vi "ADAM_scan_table.vi"() -> ()   [LabVIEW 2013]
uses:
  Anemometry/Anemometry Sub Vis/Controls/Serveds.ctl
  ADAM Client/Sub VIs/ADAM Controls/Module_type_ADAM.ctl
  ADAM Client/Sub VIs/ADAM Controls/Traverse_Level_State.ctl
  Anemometry/Anemometry Sub Vis/Controls/Post_Process.ctl
  ADAM Client/Sub VIs/ADAM Controls/Channel_State.ctl
  ADAM Client/Sub VIs/ADAM Controls/Ch_description_ADAM.ctl
  ADAM Client/Sub VIs/ADAM Controls/Function_ADAM.ctl
  ADAM Client/Sub VIs/ADAM Controls/Calib_type_ADAM.ctl
  ADAM Client/Sub VIs/ADAM Controls/Address.ctl
  ADAM_Global.vi
  Sub VI's/Channel_Description_Global.vi
  Anemometry/Anemometry Sub Vis/Globals/Meas_global.vi
  Sub VI's/Logged_Data_real_Global.vi
  Anemometry/Anemometry Sub Vis/Globals/Preference_global.vi
  Anemometry/Anemometry Sub Vis/Globals/Gas_management_global.vi
  Anemometry/Anemometry Sub Vis/Globals/Constants_global.vi
panel:
  in  "Reconfigure Gills":bool
  in  "Full Res Pathname":path
  in  "Log full Res Data":bool
  out "Duty No":u16 format="%.0b"
  in  "Save Current setup":bool=TRUE
  in  "Load setup from file":bool
  out "ADAM scan comments":string
  out "History length":i32=250
  in  "stop":bool
  out "Results":dbl[](array[numeric]) format="%.3f"
  out "Titles":string[](array[string])
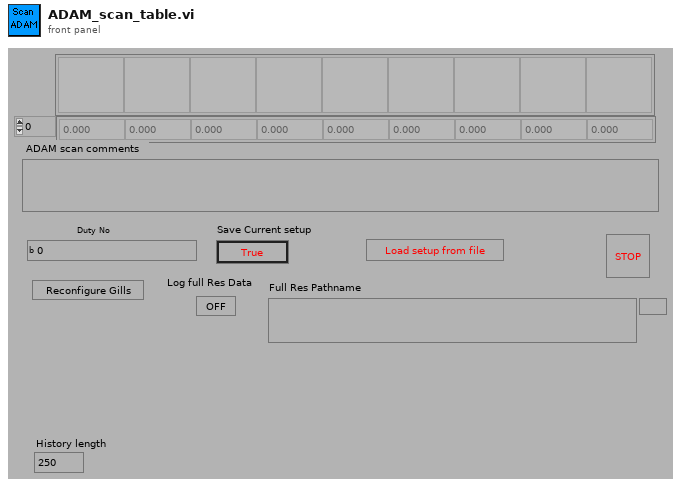
[diagram p1: front panel]
types:
  T1 = enum16{"Load ADAM setup from excel file", "Save ADAM setup to excel file"}
  T2 = typedef "Serveds.ctl" = enum16{"Read Global", "Load Global From File"}
  T3 = typedef "Module_type_ADAM.ctl" = string
  T4 = typedef "Traverse_Level_State.ctl" = enum16{"Running", "Complete"}
  T5 = typedef "Post_Process.ctl" = enum16{"Take New Data", "Post Process Raw Data File"}
  T6 = typedef "Channel_State.ctl" = enum16{"On", "Off", "Always On", "Always Off"}
  T7 = enum16{"Append to Global", "Read Global then Clear"}
  T8 = typedef "Ch_description_ADAM.ctl" = cluster{"Ch Name":string, "Type":T3, "Function":T9, "Ch State":T6, "Calibration type":T10, "A":dbl, "B":dbl, "C":dbl, "D":dbl, "Comments":string, "Address":T11, "String":string, "Duty":u16}
  T9 = typedef "Function_ADAM.ctl" = enum16{"Analogue Input", "Digital Input", "Event counter", "Event rate", "Analogue Output", "Digital Output", "Relay Output"}
  T10 = typedef "Calib_type_ADAM.ctl" = enum16{"Raw", "Bx + A", "Cx^2 + Bx + A", "Dx^3 + Cx^2 + Bx + A", "In Band", "Hi-Tec Q", "Hi-Tec M_dot", "Text"}
  T11 = typedef "Address.ctl" = cluster{"Main":i32, "Ch.":i32, "Sub":i32, "Port Name":string}
  T12 = typedef "Client_State_Cluster.ctl" = cluster{"Client Name":string, "Traverse level State":T4, "People to Email":string[], "Next Contact Time":dbl}
  T13 = typedef "ADAM_Comparitor.ctl" = cluster{"Ch to Monitor":string, "Channels to Kill":string, "Warn if Above":dbl, "Warn if Below":dbl, "Kill if Above":dbl, "Kill if Below":dbl, "Hysteresis Margin":dbl, "Averaging TIme (s)":dbl, "Warn Status":bool, "Kill Status":bool, "Extra Email addresses":string}
  T14 = typedef "Update_scan_value.ctl" = cluster{"Channel Name":string, "New Value":dbl}
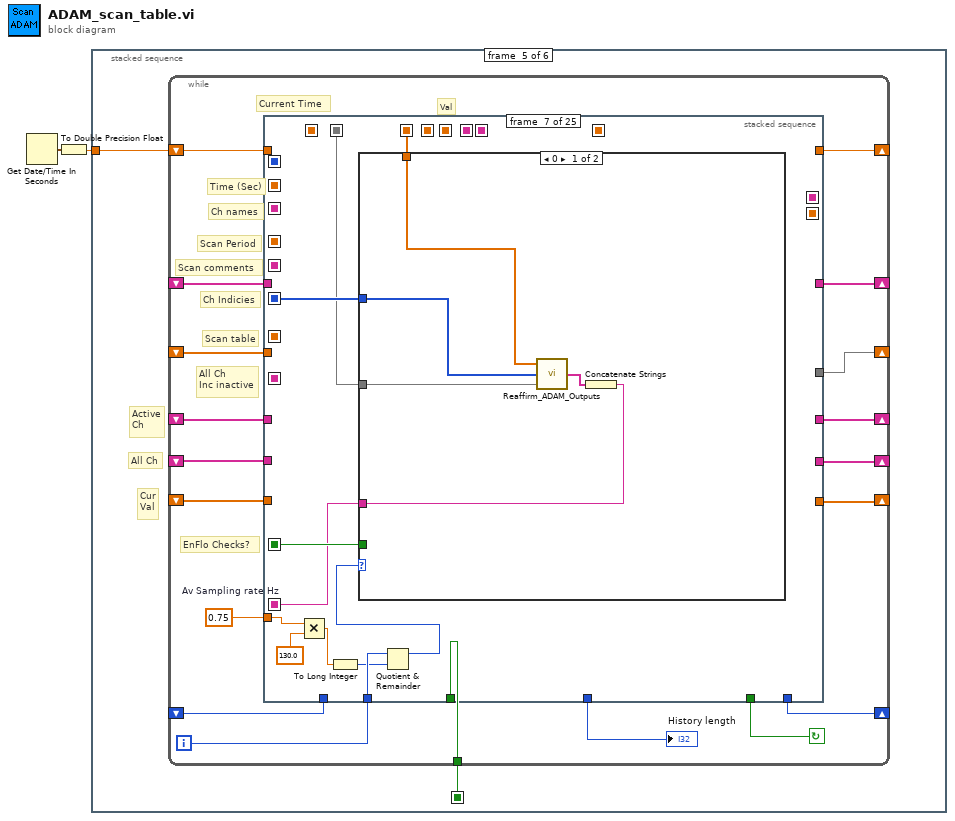
[diagram p0: block diagram]
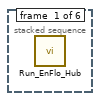
[diagram p2: hidden frame]
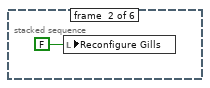
[diagram p3: hidden frame]
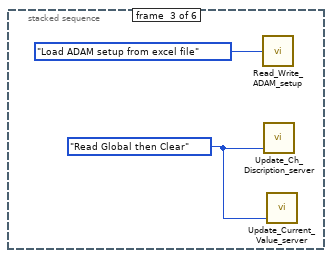
[diagram p4: hidden frame]
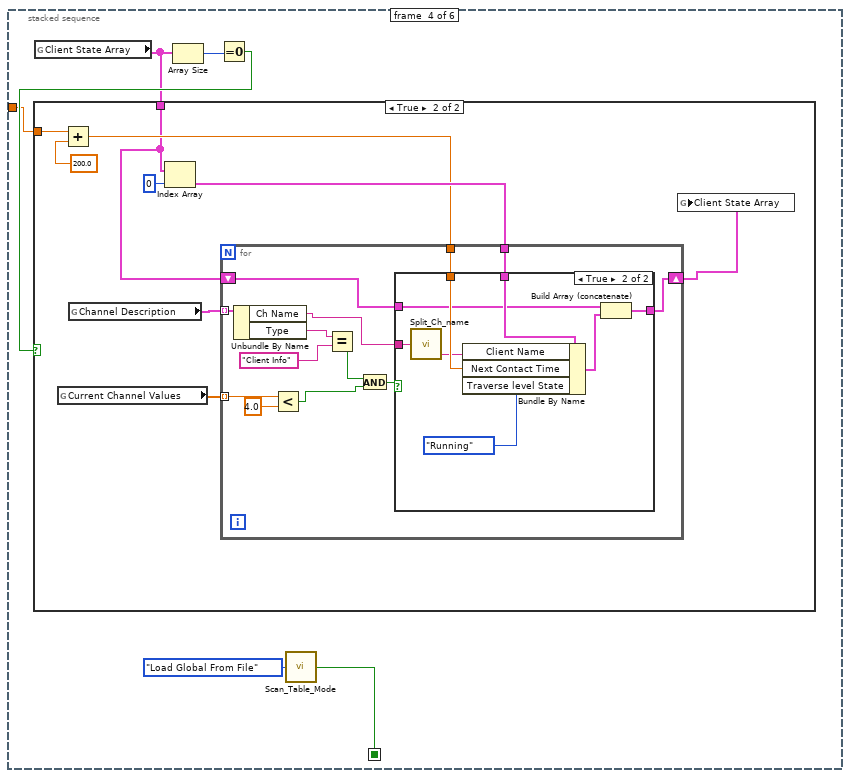
[diagram p5: hidden frame]
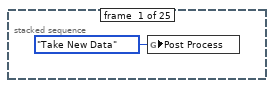
[diagram p8: hidden frame]
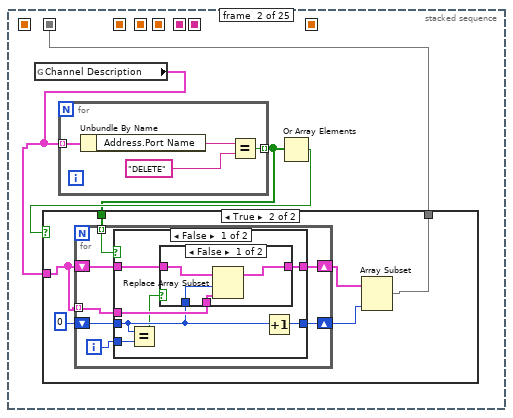
[diagram p9: hidden frame]
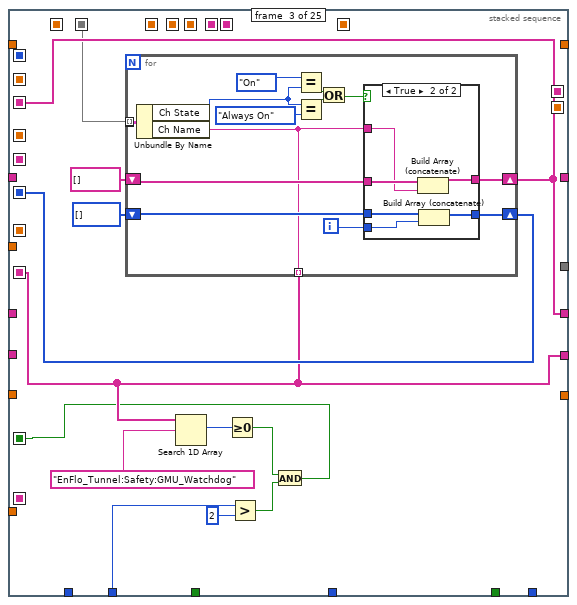
[diagram p13: hidden frame]
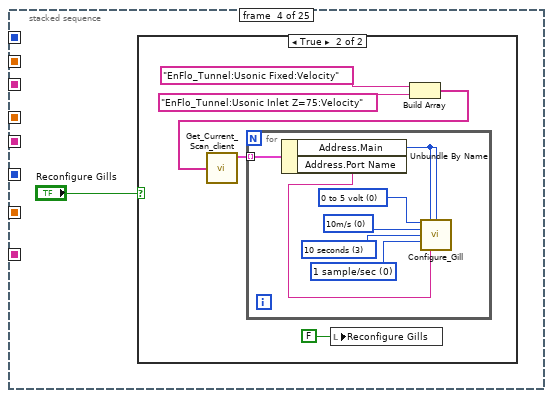
[diagram p15: hidden frame]
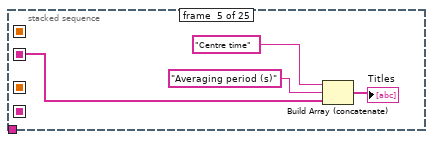
[diagram p17: hidden frame]
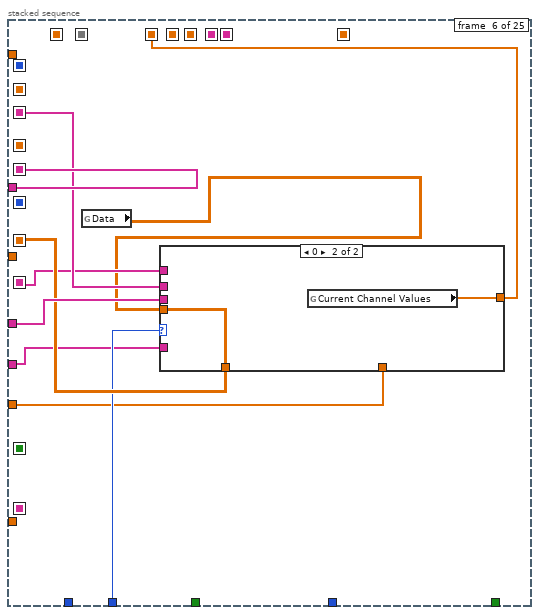
[diagram p18: hidden frame]
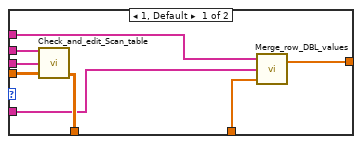
[diagram p19: hidden frame]
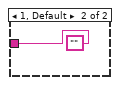
[diagram p20: hidden frame]
diagram:
  n1 = Get Date/Time In Seconds() -> (seconds since 1Jan1904=w2:timestamp)
  n2 = To Double Precision Float(number=w2) -> (double precision float=w1:dbl)
  n3 = stacked-sequence {
    seq-local: [_ _ _ w11 _ _] -> [_ _ _ _ w44 _]
    tunnel: w1 -> [_ _ _ w6 w43 _]
    frame #0 {
      n4 = call "Run_EnFlo_Hub.vi"() -> ()  [unwired: 8 out]
    }
    frame #1 {
      n5 = local write "Reconfigure Gills"(FALSE ("Reconfigure Gills")) -> ()
    }
    frame #2 {
      w4 = T7."Read Global then Clear" ("Mode")
      n6 = call "Read_Write_ADAM_setup.vi"("Mode"=T1."Load ADAM setup from excel file") -> ()  [unwired: 4 out]
      n7 = call "Update_Ch_Discription_server.vi"("Mode"=w4) -> ()  [unwired: 2 in, 1 out]
      n8 = call "Update_Current_Value_server.vi"("Mode"=w4) -> ()  [unwired: 2 in, 1 out]
    }
    frame #3 {
      n9 = global read "ADAM_Global.vi" "Client State Array"() -> (w7:T12[])
      n10 = Array Size(array=w7) -> (size(s)=w9:i32)
      n11 = Equal To 0?(x=w9) -> (x = 0?=w8:bool)
      n12 = case shown="True" w8 {
        tunnel: w7 -> [_ w13]
        tunnel: w6 -> [_ w16]
        frame False {
        }
        frame True {
          n13 = global read "ADAM_Global.vi" "Current Channel Values"() -> (w20:dbl[])
          n14 = Add(x=w16, y=200.0) -> (x+y=w14:dbl)
          n15 = global read "Channel_Description_Global.vi" "Channel Description"() -> (w19:T8[])
          n16 = Index Array(array=w13, index=0) -> (element=w17:T12)
          n17 = for {
            tunnel: w19 -> [w33] mode=indexing
            tunnel: w20 -> [w25] mode=indexing
            tunnel: w17 -> [w26]
            tunnel: w14 -> [w24]
            shift-right: [w23] -> w12
            shift-left: w13 -> [w22]
            n18 = Unbundle By Name(w33) -> ("Ch Name"=w21:string, "Type"=w30:T3)
            n19 = Less?(x=w25, y=4.0) -> (x < y?=w28:bool)
            n20 = Equal?(x=w30, y=T3 "Client Info" ("Type")) -> (x = y?=w29:bool)
            n21 = And(x=w29, y=w28) -> (x .and. y?=w27:bool)
            n22 = case shown="True" w27 {
              tunnel: w26 -> [_ w42]
              tunnel: w24 -> [_ w41]
              tunnel: [w34 w39] -> w23
              tunnel: w22 -> [w34 w38]
              tunnel: w21 -> [_ w36]
              frame False {
              }
              frame True {
                n23 = call "Split_Ch_name.vi"("Ch name"=w36) -> ("Low level"=w35:string)  [unwired: 2 out]
                n24 = Bundle By Name(cluster=w42, "Client Name"=w35, "Next Contact Time"=w41, "Traverse level State"=Traverse_Level_State."Running") -> (w37:T12)
                n25 = Build Array (concatenate)(w38, w37) -> (w39:T12[])
              }
            }
          }
          n26 = global write "ADAM_Global.vi" "Client State Array"(w12) -> ()
        }
      }
      n27 = call "Scan_Table_Mode.vi"("Mode"=Serveds."Load Global From File") -> ("Simulate Mode ?"=w11:bool)
    }
    frame #4 {
      # "Active\nCh"
      # "Cur\nVal"
      # "All Ch"
      n28 = while {
        shift-left: _ -> [w47]
        shift-right: [w46] -> _
        shift-left: _ -> [w48]
        shift-right: [w49] -> _
        shift-left: _ -> [w50]
        shift-right: [w51] -> _
        tunnel: w44 -> [w52]
        shift-left: _ -> [w55]
        shift-right: [w54] -> _
        shift-left: _ -> [w57]
        shift-right: [w58] -> _
        shift-left: _ -> [w59]
        shift-right: [w60] -> _
        shift-left: w43 -> [w61]
        shift-right: [w62] -> _
        i -> [w56]
        stop <- w63 continue-if-true
        w45 = 0.75  # Av Sampling rate Hz
        # "Current Time"
        # "EnFlo Checks?"
        # "Val"
        # "All Ch\nInc inactive"
        # "Scan comments"
        # "Scan table"
        # "Time (Sec)"
        # "Ch Indicies"
        # "Ch names"
        # "Scan Period"
        n29 = stacked-sequence {
          seq-local: [_ _ _ _ _ _ _ _ _ _ _ _ _ _ _ w315 _ _ _ _ _ _ _ _ _] -> [_ _ _ _ _ _ _ _ _ _ _ _ _ _ _ _ _ w366 w371 _ _ _ _ w449 _]
          seq-local: [_ _ _ _ _ _ _ _ w199 _ _ _ _ _ _ _ _ _ _ _ _ _ _ _ _] -> [_ _ _ _ _ _ _ _ _ _ _ _ _ _ _ _ _ _ w378 _ _ _ _ _ _]
          seq-local: [_ _ _ _ _ w158 _ _ _ _ _ _ _ _ _ _ _ _ _ _ _ _ _ _ _] -> [_ _ _ _ _ _ _ w192 _ _ _ _ _ _ _ _ _ _ w376 _ _ _ _ _ _]
          seq-local: [_ _ _ _ _ _ _ _ w203 _ _ _ _ _ _ _ _ _ _ _ _ _ _ _ _] -> [_ _ _ _ _ _ _ _ _ _ w226 _ _ _ _ _ _ _ w377 _ _ _ _ _ _]
          seq-local: [_ _ _ _ _ w161 _ _ _ _ _ _ _ _ _ _ _ _ _ _ _ _ _ _ _] -> [_ _ _ _ _ _ _ w194 _ _ _ _ _ _ _ _ _ _ _ _ w416 _ _ _ _]
          seq-local: [_ _ _ _ _ _ _ _ _ _ w224 _ _ _ _ _ _ _ _ _ _ _ _ _ _] -> [_ _ _ _ _ _ _ _ _ _ _ w243 _ _ _ _ _ _ _ _ _ _ _ _ _]
          seq-local: [_ _ w112 _ _ _ _ _ _ _ _ _ _ _ _ _ _ _ _ _ _ _ _ _ _] -> [_ _ _ _ w150 w160 _ w195 w204 _ _ _ _ _ _ _ _ _ w374 w379 _ _ _ _ _]
          seq-local: [_ _ w111 _ _ _ _ _ _ _ _ _ _ _ _ _ _ _ _ _ _ _ _ _ _] -> [_ _ _ _ _ _ w175 w190 _ _ w225 _ _ _ _ _ _ _ _ _ _ _ _ _ _]
          seq-local: [_ _ _ _ _ w154 _ _ _ _ _ _ _ _ _ _ _ _ _ _ _ _ _ _ _] -> [_ _ _ _ _ _ w173 w191 _ _ w222 _ _ _ _ _ _ _ _ _ _ _ _ _ _]
          seq-local: [_ _ _ _ _ _ _ _ _ _ w220 _ _ _ _ _ _ _ _ _ _ _ _ _ _] -> [_ _ _ _ _ _ _ _ _ _ _ w248 w277 _ _ w313 _ _ _ _ _ _ _ _ _]
          seq-local: [_ _ w107 _ _ _ _ _ _ _ _ _ _ _ _ _ _ _ _ _ _ _ _ _ _] -> [_ _ _ _ _ w156 _ w193 _ _ w221 w247 w276 _ _ w314 w339 w358 w373 _ _ _ w426 _ _]
          seq-local: [_ _ _ _ _ _ _ _ _ w206 _ _ _ _ _ _ _ _ _ _ _ _ _ _ _] -> [_ _ _ _ _ _ _ _ _ _ w219 _ _ _ _ _ _ _ _ _ _ _ _ _ _]
          seq-local: [_ w65 _ _ _ _ _ _ _ _ _ _ _ _ _ _ _ _ _ _ _ _ _ _ _] -> [_ _ w109 _ _ _ w174 w189 _ _ w218 _ _ _ _ _ _ _ _ _ _ _ _ _ _]
          seq-local: [_ _ _ _ _ _ _ _ w198 _ _ _ _ _ _ _ _ _ _ _ _ _ _ _ _] -> [_ _ _ _ _ _ _ _ _ _ _ w244 _ _ _ _ _ _ _ w381 _ _ _ _ _]
          seq-local: [_ _ _ _ _ _ _ _ _ _ _ _ _ _ _ _ _ _ w370 _ _ _ _ _ _] -> [_ _ _ _ _ _ _ _ _ _ _ _ _ _ _ _ _ _ _ w380 _ _ _ _ _]
          seq-local: [_ _ w101 _ _ _ _ _ _ _ _ _ _ _ _ _ _ _ _ _ _ _ _ _ _] -> [_ _ _ _ _ _ w182 _ w196 _ _ w246 w275 w290 w299 _ _ _ _ _ _ _ _ _ w453]
          seq-local: [_ _ _ _ _ _ _ _ _ _ _ _ _ _ _ w312 _ _ _ _ _ _ _ _ _] -> [_ _ _ _ _ _ _ _ _ _ _ _ _ _ _ _ w340 _ _ _ _ _ _ _ _]
          seq-local: [_ _ _ _ _ _ w172 _ _ _ _ _ _ _ _ _ _ _ _ _ _ _ _ _ _] -> [_ _ _ _ _ _ _ _ _ _ w217 _ _ _ _ _ _ _ _ _ _ _ _ _ _]
          seq-local: [_ _ _ _ _ _ _ _ _ _ _ _ _ _ _ w311 _ _ _ _ _ _ _ _ _] -> [_ _ _ _ _ _ _ _ _ _ _ _ _ _ _ _ w338 _ _ _ _ _ _ _ _]
          seq-local: [_ _ _ _ _ _ _ _ _ _ _ w242 _ _ _ _ _ _ _ _ _ _ _ _ _] -> [_ _ _ _ _ _ _ _ _ _ _ _ _ _ _ _ _ _ _ _ w404 _ _ _ _]
          tunnel: [_ _ _ _ _ _ _ _ _ _ _ _ _ _ _ _ _ _ _ _ _ w424 _ _ _] -> w63
          tunnel: [_ _ _ _ _ _ _ _ w198 _ _ _ _ _ _ _ _ _ _ _ _ _ _ _ _] -> w62
          tunnel: w61 -> [_ _ _ _ _ _ _ _ w200 _ _ _ _ _ _ _ _ _ _ _ _ _ _ _ _]
          tunnel: [_ _ _ _ _ _ _ _ _ _ _ _ _ _ _ _ _ _ _ _ w414 _ _ _ _] -> w60
          tunnel: w59 -> [_ _ _ _ _ w161 _ _ _ _ _ _ _ _ _ _ _ _ _ _ _ _ _ _ _]
          tunnel: [_ _ w112 _ _ _ _ _ _ _ _ _ _ _ _ _ _ _ _ _ _ _ _ _ _] -> w58
          tunnel: w57 -> [_ _ _ _ _ w159 _ _ _ _ _ _ _ _ _ _ w341 _ _ _ _ _ _ _ _]
          tunnel: w56 -> [_ _ w105 _ _ w157 w178 _ _ _ _ w245 w271 w286 w295 _ _ _ _ _ _ w422 _ _ w454]
          tunnel: w55 -> [_ _ _ _ _ _ _ _ _ _ _ _ _ _ _ _ _ w364 _ _ _ _ _ _ _]
          tunnel: [_ _ _ _ _ _ _ _ _ _ _ _ _ _ _ _ _ w360 _ _ _ _ _ _ _] -> w54
          tunnel: [_ _ _ _ _ _ _ _ _ _ _ _ _ _ _ _ _ _ w375 _ _ _ _ _ _] -> w53
          tunnel: w52 -> [_ _ _ _ _ _ _ _ _ _ w223 _ _ _ _ _ _ _ _ _ _ _ _ _ _]
          tunnel: [_ _ w107 _ _ _ _ _ _ _ _ _ _ _ _ _ _ _ _ _ _ _ _ _ _] -> w51
          tunnel: w50 -> [_ _ _ _ _ w155 _ _ _ _ _ _ _ _ _ _ _ _ _ _ _ _ _ _ _]
          tunnel: [_ _ _ _ _ _ _ _ _ _ _ _ _ _ _ _ _ _ _ _ _ _ _ w449 _] -> w49
          tunnel: w48 -> [_ _ _ _ _ w153 _ _ _ _ _ _ _ _ _ _ _ _ _ _ _ _ _ _ _]
          tunnel: w47 -> [_ _ _ _ _ _ _ _ _ w207 _ _ _ _ _ _ _ _ _ _ _ _ _ _ _]
          tunnel: [_ _ _ _ _ _ _ _ _ w208 _ _ _ _ _ _ _ _ _ _ _ _ _ _ _] -> w46
          tunnel: w45 -> [_ _ _ _ _ _ w181 _ _ _ _ _ w274 w289 w298 _ _ _ _ _ _ _ _ _ _]
          frame #0 {
            n30 = global write "Meas_global.vi" "Post Process"(Post_Process."Take New Data" ("Post Process")) -> ()
          }
          frame #1 {
            n31 = global read "Channel_Description_Global.vi" "Channel Description"() -> (w67:T8[])
            n32 = for {
              tunnel: w67 -> [w100] mode=indexing
              tunnel: [w97] -> w66 mode=indexing
              n33 = Unbundle By Name(w100) -> ("Address.Port Name"=w99:string)
              n34 = Equal?(x=w99, y="DELETE") -> (x = y?=w97:bool)
            }
            n35 = Or Array Elements(Boolean array=w66) -> (logical OR=w68:bool)
            n36 = case shown="True" w68 {
              tunnel: w67 -> [w69 w73]
              tunnel: w66 -> [_ w75]
              tunnel: [w69 w70] -> w65
              frame False {
              }
              frame True {
                n37 = for {
                  shift-right: [w82] -> w72
                  shift-left: w73 -> [w81]
                  tunnel: w75 -> [w77] mode=indexing
                  shift-right: [w80] -> w71
                  shift-left: 0 -> [w78]
                  tunnel: w73 -> [w79] mode=indexing
                  i -> [w76]
                  n38 = case shown="False" w77 {
                    tunnel: [w88 w96] -> w82
                    tunnel: w81 -> [w89 w96]
                    tunnel: [w86 w95] -> w80
                    tunnel: w78 -> [w85 w95]
                    tunnel: w79 -> [w87 _]
                    tunnel: w76 -> [w84 _]
                    frame False {
                      n39 = Equal?(x=w85, y=w84) -> (x = y?=w83:bool)
                      n40 = case shown="False" w83 {
                        tunnel: w89 -> [w93 w94]
                        tunnel: [w92 w94] -> w88
                        tunnel: w87 -> [w91 _]
                        tunnel: w85 -> [w90 _]
                        frame False {
                          n41 = Replace Array Subset(array=w93, new element=w91, index=w90) -> (w92:T8[])
                        }
                        frame True {
                        }
                      }
                      n42 = Increment(x=w85) -> (x+1=w86:i32)
                    }
                    frame True {
                    }
                  }
                }
                n43 = Array Subset(array=w72, length=w71) -> (w70:T8[])  [unwired: 1 in]
              }
            }
          }
          frame #2 {
            n44 = for {
              tunnel: [w126] -> _ mode=indexing
              shift-right: [w125] -> w112
              shift-left: string[] [] -> [w116]
              shift-right: [w122] -> w111
              shift-left: i32[] [] -> [w124]
              tunnel: [w114] -> w107 mode=indexing
              tunnel: w109 -> [w126] mode=indexing
              i -> [w123]
              n45 = Unbundle By Name(w126) -> ("Ch State"=w117:T6, "Ch Name"=w114:string)
              n46 = Equal?(x=Channel_State."On" ("Channel State"), y=w117) -> (x = y?=w119:bool)
              n47 = Equal?(x=w117, y=Channel_State."Always On" ("Channel State")) -> (x = y?=w118:bool)
              n48 = Or(x=w119, y=w118) -> (x .or. y?=w115:bool)
              n49 = case shown="True" w115 {
                tunnel: w116 -> [w127 w134]
                tunnel: w114 -> [_ w133]
                tunnel: [w127 w132] -> w125
                tunnel: w124 -> [w128 w131]
                tunnel: w123 -> [_ w130]
                tunnel: [w128 w129] -> w122
                frame False {
                }
                frame True {
                  n50 = Build Array (concatenate)(w134, w133) -> (w132:string[])
                  n51 = Build Array (concatenate)(w131, w130) -> (w129:i32[])
                }
              }
            }
            n52 = Search 1D Array(1D array=w107, element="EnFlo_Tunnel:Safety:GMU_Watchdog") -> (index of element=w106:i32)  [unwired: 1 out]
            n53 = Greater Or Equal To 0?(x=w106) -> (x >= 0?=w102:bool)
            n54 = Greater?(x=w105, y=2) -> (0:w103:bool)
            n55 = And(x=w102, y=w103) -> (x .and. y?=w101:bool)
          }
          frame #3 {
            n56 = case shown="True" "Reconfigure Gills" {
              frame False {
              }
              frame True {
                n57 = local write "Reconfigure Gills"(FALSE ("Reconfigure Gills")) -> ()
                n58 = Build Array("EnFlo_Tunnel:Usonic Fixed:Velocity", "EnFlo_Tunnel:Usonic Inlet Z=75:Velocity") -> (w138:string[])
                n59 = call "Get_Current_Scan_client.vi"("ADAM Ch Names"=w138) -> ("Ch Description Array"=w137:T8[])  [unwired: 3 out]
                n60 = for {
                  tunnel: w137 -> [w143] mode=indexing
                  w147 = u16 0 items=["1 sample/sec", "4 samples/sec"] ("Samples/sec")
                  w146 = u16 3 items=["OFF", "3 seconds", "5 seconds", "10 seconds"] ("Averaging Time")
                  w145 = u16 0 items=["10m/s", "20m/s", "30m/s", "40m/s", "50m/s", "60m/s", "70m/s"] ("Analogue O/P Scale")
                  w144 = u16 0 items=["0 to 5 volt", "+/-2.5 Volt", "4-20mA"] ("Analogue O/P Config")
                  n61 = Unbundle By Name(w143) -> ("Address.Main"=w142:i32, "Address.Port Name"=w141:string)
                  n62 = call "Configure_Gill.vi"("Analogue O/P Config"=w144, "ORIGINAL Address"=w142, "NEW Address"=w142, "Analogue O/P Scale"=w145, "Averaging Time"=w146, "Samples/sec"=w147, "Port Name"=w141) -> ()  [unwired: 9 out]
                }
              }
            }
          }
          frame #4 {
            n63 = Build Array (concatenate)("Centre time", "Averaging period (s)", w150) -> (→"Titles":string[])
          }
          frame #5 {
            n64 = global read "Logged_Data_real_Global.vi" "Data"() -> (w152:dbl[][])
            n65 = case shown="0" w157 {
              tunnel: w152 -> [w169 w171]
              tunnel: w160 -> [w166 _]
              tunnel: w159 -> [w168 _]
              tunnel: [w167 w171] -> w158
              tunnel: w156 -> [w165 _]
              tunnel: w155 -> [w164 _]
              tunnel: [w163 w170] -> w154
              tunnel: w153 -> [w162 _]
              frame 1, Default {
                n66 = call "Check_and_edit_Scan_table.vi"("2D array input"=w169, "Original Channels"=w168, "Present Channels"=w166) -> ("2D array output"=w167:dbl[][])  [unwired: 2 out]
                n67 = call "Merge_row_DBL_values.vi"("Present Row values"=w162, "Present Channels"=w164, "Desired Channels"=w165) -> ("Desired Row values"=w163:dbl[])  [unwired: 1 out]
              }
              frame 0 {
                n68 = global read "ADAM_Global.vi" "Current Channel Values"() -> (w170:dbl[])
              }
            }
          }
          frame #6 {
            n69 = Multiply(x=w181, y=130.0) -> (x*y=w179:dbl)
            n70 = To Long Integer(number=w179) -> (32bit integer=w177:i32)
            n71 = Quotient & Remainder(x=w178, y=w177) -> (x-y*floor(x/y)=w176:i32)  [unwired: 1 out]
            n72 = case shown="0" w176 {
              tunnel: w182 -> [_ _]
              tunnel: w175 -> [w186 _]
              tunnel: w174 -> [w185 _]
              tunnel: w173 -> [w184 _]
              tunnel: [w183 ""] -> w172
              frame 0 {
                n73 = call "Reaffirm_ADAM_Outputs.vi"("Channel Description"=w185, "Active Ch Indicies"=w186, "Current Channel Values"=w184) -> ("Scan Comments"=w187:string[])  [unwired: 2 out]
                n74 = Concatenate Strings(w187) -> (w183:string)
              }
              frame 1, Default {
              }
            }
          }
          frame #7 {
            n75 = global write "ADAM_Global.vi" "Active Ch names"(w195) -> ()
            n76 = global write "ADAM_Global.vi" "Scan comments"(w194) -> ()
            n77 = global write "Channel_Description_Global.vi" "Channel Description"(w189) -> ()
            n78 = global write "ADAM_Global.vi" "Active Ch Indicies"(w190) -> ()
            n79 = global write "ADAM_Global.vi" "All Ch names"(w193) -> ()
            n80 = global write "Logged_Data_real_Global.vi" "Data"(w192) -> ()
            n81 = global write "ADAM_Global.vi" "Current Channel Values"(w191) -> ()
          }
          frame #8 {
            n82 = case shown="True" w196 {
              tunnel: w204 -> [_ w205]
              frame False {
              }
              frame True {
                n83 = call "Gas_Status_panel.vi"("Ch names"=w205) -> ()  [unwired: 15 out]
              }
            }
            n84 = Get Date/Time In Seconds() -> (seconds since 1Jan1904=w197:timestamp)
            n85 = To Double Precision Float(number=w197) -> (double precision float=w198:dbl)
            n86 = Subtract(x=w198, y=w200) -> (x-y=w203:dbl)
            n87 = Divide(x=w203, y=2.0) -> (x/y=w201:dbl)
            n88 = Add(x=w201, y=w200) -> (x+y=w199:dbl)
          }
          frame #9 {
            n89 = Equal To 0?(x=w207) -> (x = 0?=w211:bool)
            n90 = Equal?(x=u16 32768, y=w207) -> (x = y?=w210:bool)
            n91 = Select(t=u16 1, s=w211, f=w207) -> (s? t:f=w206:u16)
            "Duty No" <- w206
            n92 = case shown="False" w210 {
              tunnel: [w213 u16 0] -> w208
              tunnel: w206 -> [w215 _]
              frame False {
                n93 = Multiply(x=u16 2, y=w215) -> (x*y=w213:u16)
              }
              frame True {
              }
            }
          }
          frame #10 {
            n94 = for {
              tunnel: w218 -> [w233]
              tunnel: w226 -> [w241]
              shift-right: [w239] -> w220
              shift-left: w222 -> [w237]
              tunnel: w221 -> [w238]
              shift-right: [w234] -> w224
              shift-left: w217 -> [w236]
              tunnel: w225 -> [w228] mode=indexing
              tunnel: w222 -> [w230]
              tunnel: w223 -> [w231]
              tunnel: w219 -> [w227]
              n95 = Index Array(array=w230, index=w228) -> (element=w229:dbl)
              n96 = Index Array(array=w233, index=w228) -> (element=w232:T8)
              n97 = call "Adam_Ch_Input_Output.vi"("Simulate"=w231, "Duty No"=w227, "Previuos Scan Value"=w229, "Ch values"=w237, "Scan Period"=w241, "Ch Discription"=w232, "Ch names"=w238) -> ("Scan comment"=w235:string, "Calibrated units"=w240:dbl)  [unwired: 1 in, 2 out]
              n98 = Concatenate Strings(w236, w235) -> (w234:string)
              n99 = Replace Array Subset(array=w237, new element=w240, index=w228) -> (w239:dbl[])
            }
          }
          frame #11 {
            n100 = case shown="True" w246 {
              tunnel: w248 -> [_ w255]
              tunnel: w247 -> [_ w254]
              tunnel: w245 -> [_ w253]
              tunnel: w244 -> [_ w263]
              tunnel: w243 -> [w250 w252]
              tunnel: [w250 w260] -> w242
              frame False {
              }
              frame True {
                n101 = global read "ADAM_Global.vi" "Comparitor Array"() -> (w259:T13[])
                n102 = for {
                  tunnel: w259 -> [w268] mode=indexing
                  tunnel: [w267] -> w258 mode=indexing
                  tunnel: w255 -> [w266]
                  tunnel: w254 -> [w265]
                  tunnel: [w264] -> w257 mode=indexing
                  n103 = call "ADAM_Comparitor.vi"("Comparator Info"=w268, "Ch names"=w265, "Present scan array"=w266) -> ("Comparator Info Out"=w267:T13, "Scan comment"=w264:string)  [unwired: 1 in]
                }
                n104 = call "LDA1_Safety.vi"("Adam Loop Count"=w253, "Ch Names"=w254, "Values"=w255) -> ("Scan comment"=w251:string)
                n105 = call "LDA2_Safety.vi"("Adam Loop Count"=w253, "Ch Names"=w254, "Values"=w255) -> ("Scan comment"=w256:string)
                n106 = call "Safety_Check.vi"("Adam Loop Count"=w253, "Ch Names"=w254, "Values"=w255) -> ("Scan comment"=w262:string)
                n107 = call "Check_Aero_Tunnel_on_Server.vi"("Values"=w255, "Ch Names"=w254, "Current Time"=w263, "Adam Loop Count"=w253) -> ("Scan comment"=w261:string)  [unwired: 2 in]
                n108 = global write "ADAM_Global.vi" "Comparitor Array"(w258) -> ()
                n109 = Concatenate Strings(w252, w251, w256, w262, w261, w257) -> (w260:string)
              }
            }
            n110 = property on="Results" class="Arr (strict)"() -> ("Index Values"=w249:u32[])  [unwired: 2 in, 2 out]
            n111 = property on="Titles" class="Arr (strict)"("Index Values"=w249) -> ()  [unwired: 2 in, 2 out]
          }
          frame #12 {
            n112 = Multiply(x=w274, y=60.0) -> (x*y=w272:dbl)
            n113 = To Long Integer(number=w272) -> (32bit integer=w270:i32)
            n114 = Quotient & Remainder(x=w271, y=w270) -> (x-y*floor(x/y)=w269:i32)  [unwired: 1 out]
            n115 = case shown="0" w269 {
              tunnel: w277 -> [w280 _]
              tunnel: w276 -> [w279 _]
              tunnel: w275 -> [w278 _]
              frame 0 {
                n116 = case shown="True" w278 {
                  tunnel: w280 -> [_ w283]
                  tunnel: w279 -> [_ w282]
                  frame False {
                  }
                  frame True {
                    w281 = TRUE  # Set Watchdogs
                    n117 = call "Do_Every_minute.vi"("Ch Names"=w282, "Values"=w283) -> ()  [unwired: 1 out]
                    n118 = call "Set_Adam_Watchdogs.vi"("Set Watchdogs"=w281) -> ()  [unwired: 1 out]
                  }
                }
              }
              frame 1, Default {
              }
            }
          }
          frame #13 {
            n119 = Multiply(x=w289, y=100.0) -> (x*y=w287:dbl)
            n120 = To Long Integer(number=w287) -> (32bit integer=w285:i32)
            n121 = Quotient & Remainder(x=w286, y=w285) -> (x-y*floor(x/y)=w284:i32)  [unwired: 1 out]
            n122 = case shown="0" w284 {
              tunnel: w290 -> [w291 _]
              frame 0 {
                n123 = case shown="True" w291 {
                  frame False {
                  }
                  frame True {
                    w292 = TRUE  # Set Watchdogs
                    n124 = call "Set_Adam_Watchdogs.vi"("Set Watchdogs"=w292) -> ()  [unwired: 1 out]
                  }
                }
              }
              frame 1, Default {
              }
            }
          }
          frame #14 {
            n125 = Multiply(x=w298, y=55.0) -> (x*y=w296:dbl)
            n126 = To Long Integer(number=w296) -> (32bit integer=w294:i32)
            n127 = Quotient & Remainder(x=w295, y=w294) -> (x-y*floor(x/y)=w293:i32)  [unwired: 1 out]
            n128 = case shown="0" w293 {
              tunnel: w299 -> [_ _]
              frame 0 {
                n129 = case shown="True" "Save Current setup" {
                  tunnel: [FALSE w303] -> w300
                  frame False {
                  }
                  frame True {
                    n130 = Get Date/Time In Seconds() -> (seconds since 1Jan1904=w305:timestamp)
                    n131 = global read "ADAM_Global.vi" "Network Last checked"() -> (w309:dbl)
                    n132 = To Double Precision Float(number=w305) -> (double precision float=w304:dbl)
                    n133 = Subtract(x=w309, y=w304) -> (x-y=w308:dbl)
                    n134 = Absolute Value(x=w308) -> (abs(x)=w307:dbl)
                    n135 = Less?(x=w307, y=1.5) -> (x < y?=w303:bool)
                  }
                }
                n136 = case shown="True" w300 {
                  frame False {
                  }
                  frame True {
                    n137 = call "Read_Write_ADAM_setup.vi"("Mode"=T1."Save ADAM setup to excel file") -> ()  [unwired: 4 out]
                  }
                }
              }
              frame 1, Default {
              }
            }
          }
          frame #15 {
            n138 = call "Update_Current_Value_server.vi"("Mode"=T7."Read Global then Clear") -> ("Update array out"=w317:T14[])  [unwired: 2 in]
            n139 = for {
              tunnel: w314 -> [w325]
              tunnel: w317 -> [w320] mode=indexing
              shift-right: [w323] -> w315
              shift-left: w313 -> [w324]
              tunnel: [w319] -> w312 mode=indexing
              tunnel: [w318] -> w311 mode=indexing
              n140 = Unbundle By Name(w320) -> ("Channel Name"=w319:string, "New Value"=w318:dbl)
              n141 = Search 1D Array(1D array=w325, element=w319) -> (index of element=w322:i32)  [unwired: 1 out]
              n142 = Less Than 0?(x=w322) -> (x < 0?=w321:bool)
              n143 = case shown="True" w321 {
                tunnel: w319 -> [_ w326]
                tunnel: w320 -> [_ w331]
                frame False {
                }
                frame True {
                  n144 = global read "ADAM_Global.vi" "Update Current Value"() -> (w330:T14[])
                  n145 = call "Check_Ch_Name_colons.vi"("No of Colons"=2, "Ch Name in"=w326) -> ("Ch Name out"=w327:string)
                  n146 = Bundle By Name(cluster=T8 {"Ch Name"="", "Type"="Hold Value", "Function"=enum."Analogue Input", "Ch State"=enum."On", "Calibration type"=enum."Raw", "A"=0.0, "B"=0.0, "C"=0.0, "D"=0.0, "Comments"="", "Address"={"Main"=0, "Ch."=0, "Sub"=0, "Port Name"=""}, "String"="", "Duty"=0} ("Ch Description"), "Ch Name"=w327, "Type"=T3 "Hold Value") -> (w335:T8)
                  n147 = Build Array (concatenate)(w330, w331) -> (w329:T14[])
                  n148 = global write "ADAM_Global.vi" "Update Current Value"(w329) -> ()
                  n149 = global read "Preference_global.vi" "Rig Setup"() -> (w333:string)
                  n150 = Build Array(w335) -> (w334:T8[])
                  n151 = call "Update_Ch_Discription_server.vi"("Mode"=T7."Append to Global", "Client HD name"=w333, "Channels to update In"=w334) -> ()  [unwired: 1 out]
                }
              }
              n152 = Replace Array Subset(array=w324, new element=w318, index=w322) -> (w323:dbl[])
            }
          }
          frame #16 {
            n153 = for {
              tunnel: w341 -> [w349]
              tunnel: w340 -> [w347] mode=indexing
              tunnel: w339 -> [w348]
              tunnel: w338 -> [w345] mode=indexing
              n154 = Search 1D Array(1D array=w349, element=w347) -> (index of element=w346:i32)  [unwired: 1 out]
              n155 = Less Than 0?(x=w346) -> (x < 0?=w344:bool)
              n156 = Not Equal To 0?(x=w345) -> (x != 0?=w343:bool)
              n157 = And(x=w343, y=w344) -> (x .and. y?=w342:bool)
              n158 = case shown="True" w342 {
                tunnel: w348 -> [_ w357]
                tunnel: w347 -> [_ w356]
                frame False {
                }
                frame True {
                  n159 = Search 1D Array(1D array=w357, element=w356) -> (index of element=w351:i32)  [unwired: 1 out]
                  n160 = global read "Channel_Description_Global.vi" "Channel Description"() -> (w352:T8[])
                  n161 = Index Array(array=w352, index=w351) -> (element=w355:T8)
                  n162 = Bundle By Name(cluster=w355, "Ch State"=Channel_State."On") -> (w353:T8)
                  n163 = Replace Array Subset(array=w352, new element=w353, index=w351) -> (w350:T8[])
                  n164 = global write "Channel_Description_Global.vi" "Channel Description"(w350) -> ()
                }
              }
            }
          }
          frame #17 {
            n165 = Search 1D Array(1D array=w358, element="GMU:Source:Release Temp") -> (index of element=w365:i32)  [unwired: 1 out]
            n166 = Index Array(array=w366, index=w365) -> (element=w363:dbl)
            n167 = Build Array (concatenate)(w363, w364) -> (w362:dbl[])
            n168 = Array Subset(array=w362, length=10 ("Array Length")) -> (w360:dbl[])  [unwired: 1 in]
            n169 = call "Mean_fr_NaN_data.vi"("Data"=w360) -> ("Mean value"=w359:dbl)  [unwired: 1 out]
            n170 = global write "Gas_management_global.vi" "Release temp (deg C)"(w359) -> ()
          }
          frame #18 {
            w368 = 250000  # Table size
            n171 = call "Merge_row_DBL_values.vi"("Present Row values"=w371, "Present Channels"=w373, "Desired Channels"=w374) -> ("Desired Row values"=w372:dbl[])  [unwired: 1 out]
            n172 = Build Array (concatenate)(w378, w377, w372) -> (w370:dbl[])
            "Results" <- w370
            n173 = call "Manipulate_Table.vi"("Table size"=w368, "Latest Row"=w370, "Table Input"=w376) -> ("History length"=w375:i32, "Table Output"=w369:dbl[][])  [unwired: 1 out]
            n174 = global write "Logged_Data_real_Global.vi" "Data"(w369) -> ()
          }
          frame #19 {
            n175 = case shown="True" "Log full Res Data" {
              tunnel: w381 -> [_ w394]
              tunnel: w380 -> [_ w393]
              tunnel: w379 -> [_ w392]
              frame False {
              }
              frame True {
                n176 = Build Array (concatenate)(w394, w393) -> (w391:dbl[])
                n177 = Number To Fractional String(number=w391) -> (F-format string=w389:string[])  [unwired: 3 out]
                n178 = call "Does_file_exist_(simple).vi"("Pathname"="Full Res Pathname") -> ("exists?"=w388:bool)
                n179 = Build Array (concatenate)("Current time", "Centre Time", "Averaging period (s)", w392) -> (w390:string[])
                n180 = case shown="False" w388 {
                  tunnel: w390 -> [w400 _]
                  tunnel: w389 -> [w399 w401]
                  tunnel: [w396 w402] -> w384
                  frame False {
                    n181 = Build Array(w400, w399) -> (w397:string[][])
                    n182 = Array To Spreadsheet String(array=w397, 3:"%s" ("format string")) -> (spreadsheet string=w396:string)  [unwired: 1 out]
                  }
                  frame True {
                    n183 = Array To Spreadsheet String(array=w401, 3:"%s" ("format string")) -> (spreadsheet string=w402:string)  [unwired: 1 out]
                  }
                }
                n184 = call "Write_File_Simple.vi"("append to file? (new file:F)"=TRUE, "character string"=w384, "file path"="Full Res Pathname") -> ()  [unwired: 2 out]
              }
            }
          }
          frame #20 {
            w412 = 150 ("length")
            w413 = 50  # History length
            n185 = String Subset(string=w404, length (rest)=w412) -> (substring=w406:string)  [unwired: 1 out]
            n186 = String Length(string=w406) -> (length=w411:i32)
            n187 = Equal?(x=w412, y=w411) -> (x = y?=w410:bool)
            n188 = Select(t=" Clipped ", s=w410, f="") -> (s? t:f=w407:string)
            n189 = Concatenate Strings(w407, w406) -> (w405:string)
            n190 = Build Array (concatenate)(w416, w405) -> (w415:string[])
            n191 = Array Size(array=w415) -> (size(s)=w418:i32)
            n192 = Subtract(x=w418, y=w413) -> (x-y=w417:i32)
            n193 = Array Subset(array=w415, index=w417) -> (w414:string[])  [unwired: 1 in]
            "ADAM scan comments" <- w404
          }
          frame #21 {
            n194 = Format Into String(format string="%s %d %s" ("Format String"), "\nScan No " ("Header message"), w422, "\r\n") -> (resulting string=w421:string)  [unwired: 2 in, 1 out]
            n195 = call "Write_out_serial_log.vi"("Header message"=w421) -> ()
            n196 = Not(x="stop") -> (.not. x?=w424:bool)
          }
          frame #22 {
            n197 = call "Update_Ch_Discription_server.vi"("Mode"=T7."Read Global then Clear") -> ("Channels to update Out"=w427:T8[])  [unwired: 2 in]
            n198 = Array Size(array=w427) -> (size(s)=w429:i32)
            n199 = Equal To 0?(x=w429) -> (x = 0?=w428:bool)
            n200 = case shown="False" w428 {
              tunnel: w426 -> [w434 _]
              tunnel: w427 -> [w433 _]
              frame False {
                n201 = global read "Channel_Description_Global.vi" "Channel Description"() -> (w432:T8[])
                n202 = for {
                  tunnel: w434 -> [w441]
                  tunnel: w433 -> [w438] mode=indexing
                  shift-right: [w437] -> w431
                  shift-left: w432 -> [w440]
                  n203 = Unbundle By Name(w438) -> ("Ch Name"=w439:string)
                  n204 = Search 1D Array(1D array=w441, element=w439) -> (index of element=w435:i32)  [unwired: 1 out]
                  n205 = Less Than 0?(x=w435) -> (x < 0?=w436:bool)
                  n206 = case shown="False" w436 {
                    tunnel: w440 -> [w445 w448]
                    tunnel: w438 -> [w444 w446]
                    tunnel: [w443 w447] -> w437
                    tunnel: w435 -> [w442 _]
                    frame False {
                      n207 = Replace Array Subset(array=w445, new element=w444, index=w442) -> (w443:T8[])
                    }
                    frame True {
                      n208 = Build Array (concatenate)(w448, w446) -> (w447:T8[])
                    }
                  }
                }
                n209 = global write "Channel_Description_Global.vi" "Channel Description"(w431) -> ()
              }
              frame True {
              }
            }
          }
          frame #23 {
            n210 = case shown="True" "Load setup from file" {
              frame False {
              }
              frame True {
                n211 = local write "Save Current setup"(TRUE ("Save Current setup")) -> ()
                n212 = call "Read_Write_ADAM_setup.vi"("Mode"=T1."Load ADAM setup from excel file") -> ()  [unwired: 4 out]
              }
            }
          }
          frame #24 {
            n213 = case shown="0" w454 {
              tunnel: w453 -> [_ _]
              frame 0 {
                n214 = global read "Constants_global.vi" "EnFlo SW Folder"() -> (w459:path)
                n215 = Build Path(base path=w459, name or relative path=path "ADAM Client/ADAM client VIs/Plot_Server_Data.vi") -> (appended path=w456:path)
                n216 = call "Load_Comparitor_Cluster.vi"() -> ()  [unwired: 12 in]
                n217 = Build Path(base path=w459, name or relative path=path "ADAM Server/Log_ADAM_scan_table.vi") -> (appended path=w457:path)
                n218 = Build Array(w457, w456) -> (w455:path[])
                n219 = for {
                  tunnel: w455 -> [w461] mode=indexing
                  n220 = Open VI Reference(vi path=w461) -> (vi reference=w465:refnum<vi>, error out=w464:errorcluster)  [unwired: 2 in, 3 out]
                  n221 = property class="VI"(reference=w465, error in=w464, "Front Panel Window:Open"=TRUE) -> (reference out=w462:refnum<vi>, error out=w463:errorcluster)
                  n222 = invoke class="VI" method="Run VI"(reference=w462, error in=w463, "Wait until done"=FALSE) -> (reference out=w469:refnum<vi>, error out=w468:errorcluster)  [unwired: 2 in, 3 out]
                  n223 = Close Reference(reference=w469, error in (no error)=w468) -> ()  [unwired: 1 out]
                }
              }
              frame 1, Default {
              }
            }
          }
        }
        "History length" <- w53
      }
    }
    frame #5 {
      w470 = FALSE  # Set Watchdogs
      n224 = call "Set_Adam_Watchdogs.vi"("Set Watchdogs"=w470) -> ()  [unwired: 1 out]
      n225 = call "Read_Write_ADAM_setup.vi"("Mode"=T1."Save ADAM setup to excel file") -> ()  [unwired: 4 out]
    }
  }
